vi "matrix_handling.vi"() -> ()   [LabVIEW 2016]
uses:
  <vilib>/Analysis/Matrix/Datatypes/ComplexMatrix.ctl
  <vilib>/Math Plots/3D Math Plots/3D Surface/3D Surface XCtrl/3D Surface.xctl
  <vilib>/Analysis/2dsp.llb/2D Real FFT.vi
  <vilib>/Analysis/2dsp.llb/2D Inverse Complex FFT.vi
  <vilib>/Analysis/Matrix/Numeric/Conversions/Array To Matrix - CA.vi
  <vilib>/Analysis/Matrix/Numeric/Conversions/Array To Matrix - RA2.vi
  <vilib>/Analysis/Matrix/Numeric/Complex/Cartesian To Complex - RM,RM.vi
  <vilib>/Analysis/Matrix/Numeric/Multiply/Multiply - CM,CM.vi
  <vilib>/Math Plots/3D Math Plots/3D Surface/3D Surface Datatype/Public/Plot Helper (Vector).vi
  <vilib>/Analysis/Matrix/NI_Matrix.lvlib
  <vilib>/Analysis/NI_AALPro.lvlib
  <vilib>/Math Plots/3D Math Plots/3D Surface/3D Surface Datatype/3D Surface Datatype.lvclass
panel:
  out "X":cdb[][](array[numeric])
  out "3D Surface":refnum<class "3D Plot Datatype.lvclass">[](xcontrol)
  out "Reshaped":T1
  out "Matrix 16x400":T1
  in  "error in (no error)":errorcluster
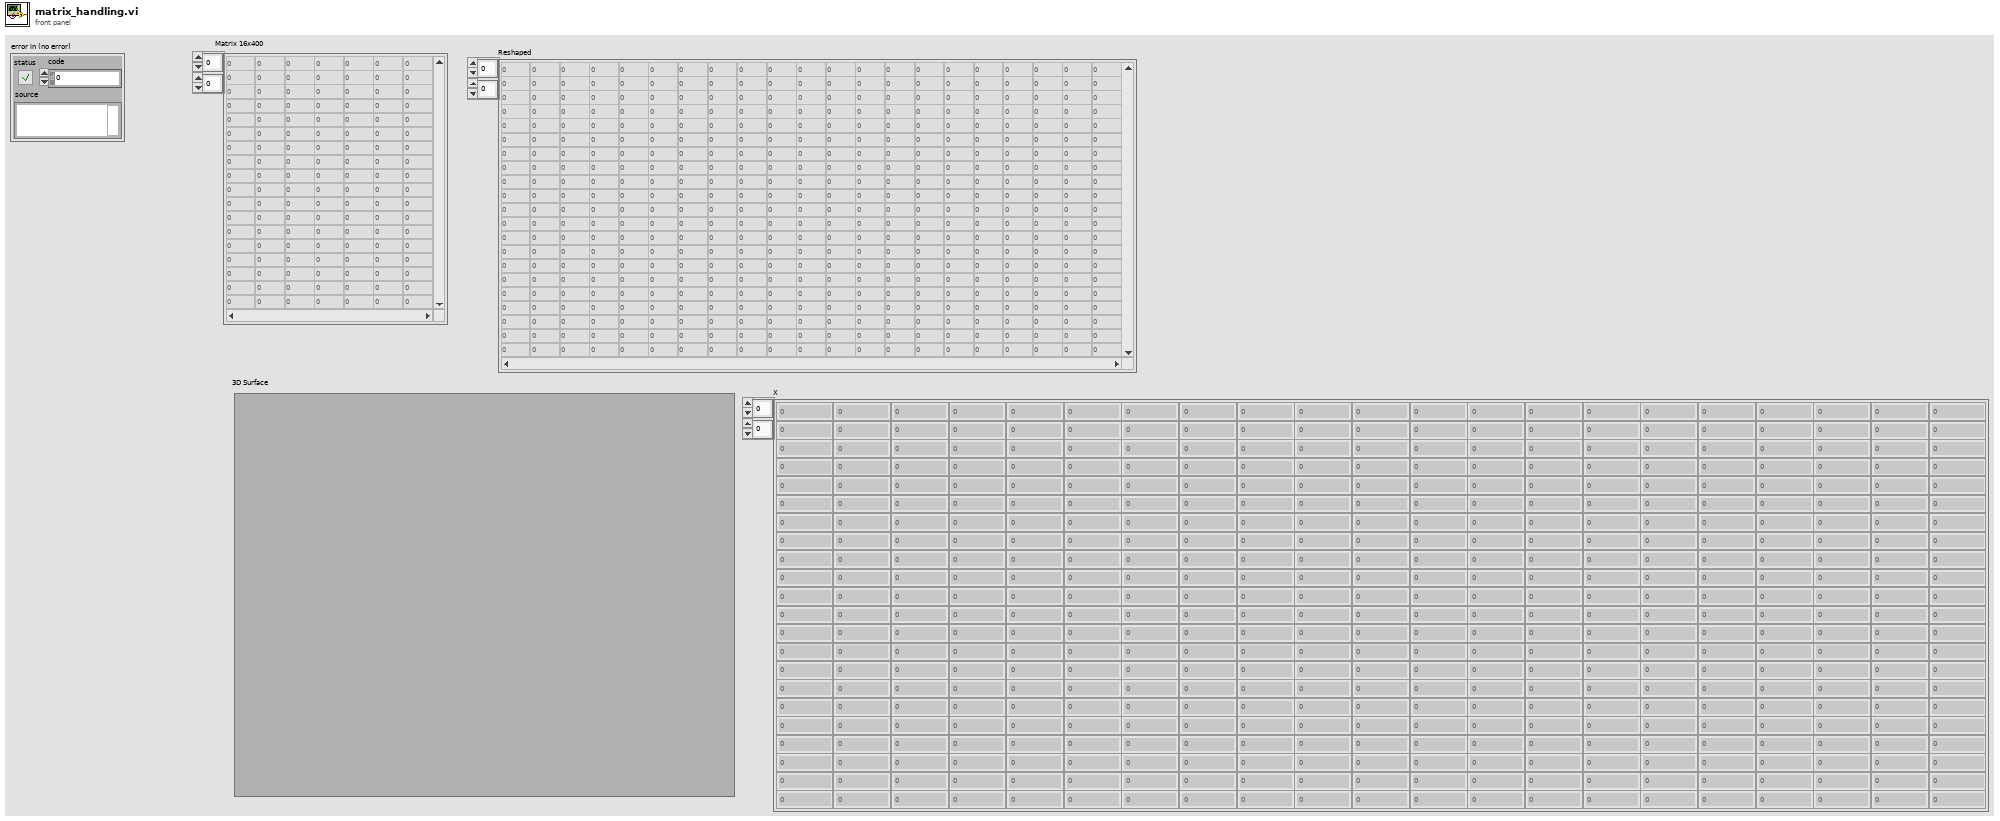
[diagram p1: front panel]
types:
  T1 = typedef "NI_Matrix.lvlib/ComplexMatrix.ctl" = cdb[][]
  T2 = enum16{"open", "replace", "create", "open or create", "replace or create", "replace or create with confirmation"}
  T3 = typedef "NI_Matrix.lvlib/RealMatrix.ctl" = dbl[][]
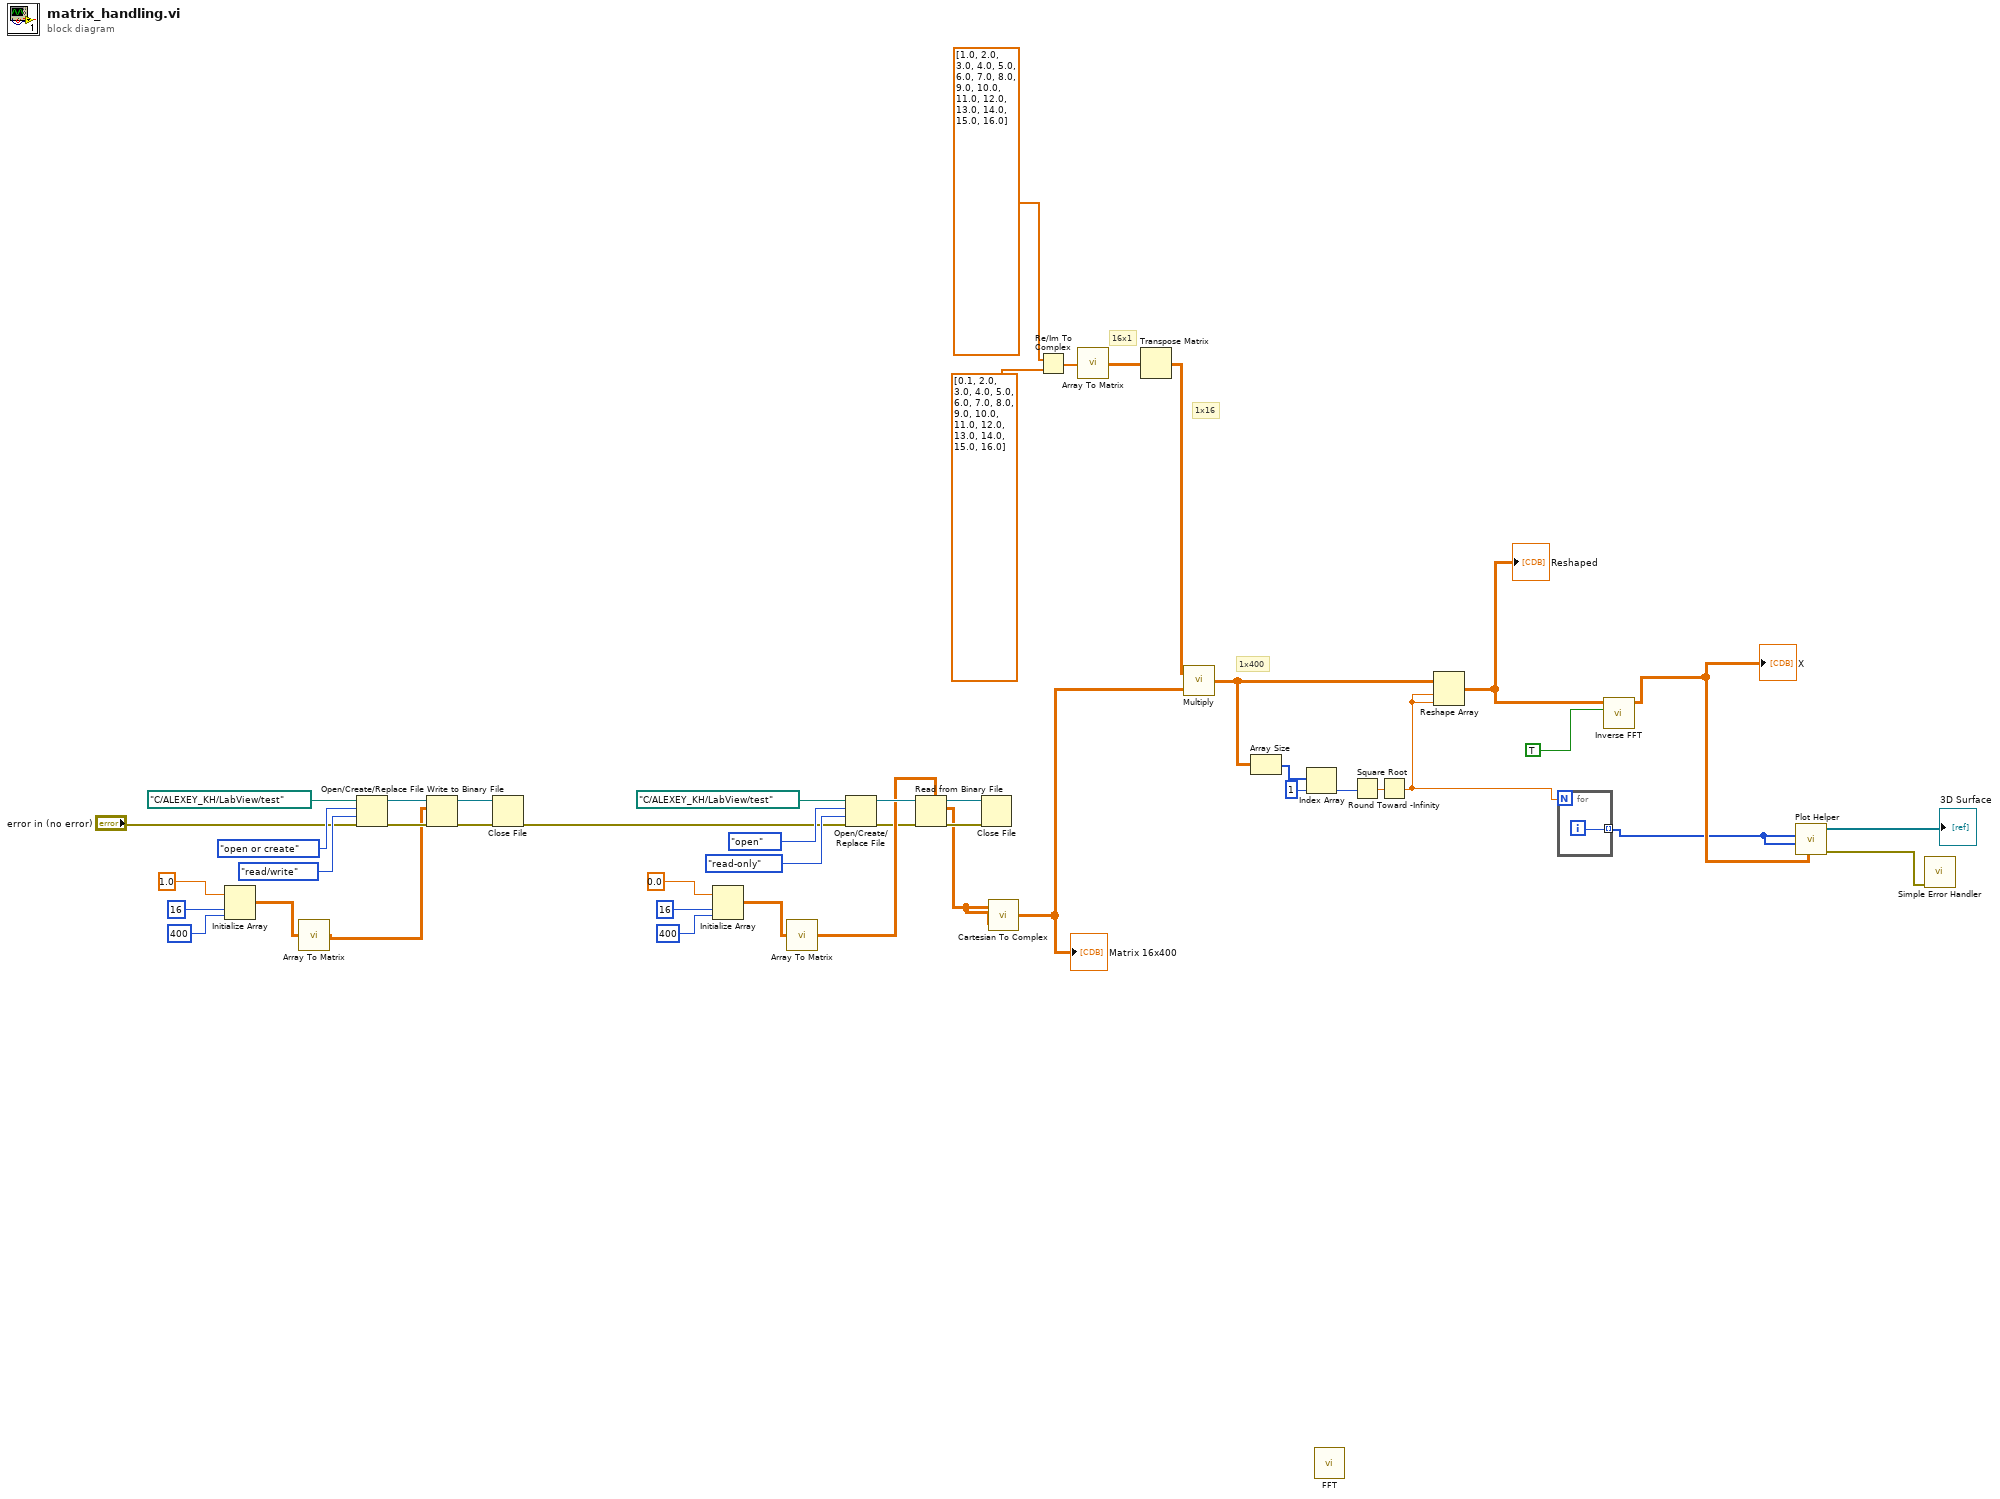
[diagram p0: block diagram]
diagram:
  # "1x400"
  # "16x1"
  # "1x16"
  n1 = Initialize Array(1.0 ("element"), 16 ("dimension size"), 400 ("dimension size")) -> (w20:dbl[][])
  n2 = call-poly <vilib>:"Array To Matrix.vi"("Real 2D Array"=w20) -> ("Real Matrix"=w9:T3)
  n3 = Open/Create/Replace File(file path (use dialog)=path "C:/ALEXEY_KH/LabView/test" ("file (use dialog)"), error in="error in (no error)", operation (0:open)=T2."open or create", access (0:read/write)=enum16{"read/write", "read-only", "write-only"}."read/write") -> (refnum out=w19:refnum<file>, error out=w28:errorcluster)  [unwired: 2 in, 1 out]
  n4 = Write to Binary File(file (use dialog)=w19, data=w9, error in=w28) -> (refnum out=w26:refnum<file>, error out=w27:errorcluster)  [unwired: 3 in, 1 out]
  n5 = Close File(refnum=w26, error in=w27) -> (error out=w11:errorcluster)  [unwired: 1 out]
  n6 = Initialize Array(0.0 ("element"), 16 ("dimension size"), 400 ("dimension size")) -> (w40:dbl[][])
  n7 = call-poly <vilib>:"Array To Matrix.vi"("Real 2D Array"=w40) -> ("Real Matrix"=w36:T3)
  n8 = Open/Create/Replace File(file path (use dialog)=path "C:/ALEXEY_KH/LabView/test" ("file (use dialog)"), error in=w11, operation (0:open)=T2."open", access (0:read/write)=enum16{"read/write", "read-only", "write-only"}."read-only") -> (refnum out=w41:refnum<file>, error out=w31:errorcluster)  [unwired: 2 in, 1 out]
  n9 = Read from Binary File(5:w36, 8:w31, 11:w41) -> (0:w32:errorcluster, 2:w15:T3, 3:w33:refnum<file>)  [unwired: 3 in, 1 out]
  n10 = Close File(refnum=w33, error in=w32) -> ()  [unwired: 2 out]
  n11 = call-poly <vilib>:"Cartesian To Complex.vi"("Real Matrix I"=w15, "Real Matrix R"=w15) -> ("R + Ii"=w17:T1)
  "Matrix 16x400" <- w17
  n12 = Re/Im To Complex(1:dbl[] [0.1, 2.0, 3.0, 4.0, 5.0, 6.0, 7.0, 8.0, 9.0, 10.0, 11.0, 12.0, 13.0, 14.0, 15.0, 16.0], 2:dbl[] [1.0, 2.0, 3.0, 4.0, 5.0, 6.0, 7.0, 8.0, 9.0, 10.0, 11.0, 12.0, 13.0, 14.0, 15.0, 16.0]) -> (0:w43:cdb[])
  n13 = call-poly <vilib>:"Array To Matrix.vi"("Complex 1D Array"=w43) -> ("Complex Matrix (Column Vector)"=w30:T1)
  n14 = Transpose Matrix(1:w30) -> (0:w29:T1)
  n15 = call-poly <vilib>:"Multiply.vi"("Complex Matrix B"=w17, "Complex Matrix A"=w29) -> ("A * B"=w14:T1)
  n16 = Array Size(array=w14) -> (size(s)=w13:i32[])
  n17 = Index Array(array=w13, index=1) -> (element=w8:i32)
  n18 = call-poly <vilib>:"FFT.vi"() -> ()  [unwired: 10 in, 2 out]
  n19 = Square Root(x=w8) -> (sqrt(x)=w3:dbl)
  n20 = Round Toward -Infinity(1:w3) -> (0:w1:dbl)
  n21 = Reshape Array(w14, w1, w1) -> (w7:T1)
  "Reshaped" <- w7
  n22 = for {
    N: w1 -> [_]
    tunnel: [w46] -> w2 mode=indexing
    i -> [w46]
  }
  n23 = call-poly <vilib>:"Inverse FFT.vi"("shift?"=TRUE, "FFT {x}"=w7) -> ("X"=w4:cdb[][])  [unwired: 8 in, 1 out]
  "X" <- w4
  n24 = call-poly <vilib>:"Plot Helper.vi"("z matrix"=w4, "y vector"=w2, "x vector"=w2) -> ("error out"=w5:errorcluster, "3D Plot lvclass Array out"=→"3D Surface":refnum<class "3D Plot Datatype.lvclass">[])  [unwired: 4 in, 3 out]
  n25 = call <vilib>:"Simple Error Handler.vi"("error in (no error)"=w5) -> ()  [unwired: 4 in, 5 out]
